vi "Write Numeric to CSV File.vi"(8 "error in (no error)":errorcluster, 9 "Time String":string, 10 "Numeric":dbl, 11 "Byte Stream File in":refnum<file>) -> (0 "error out":errorcluster, 2 "Numeric Return":dbl, 3 "Byte Stream File out":refnum<file>)   [LabVIEW 2021]
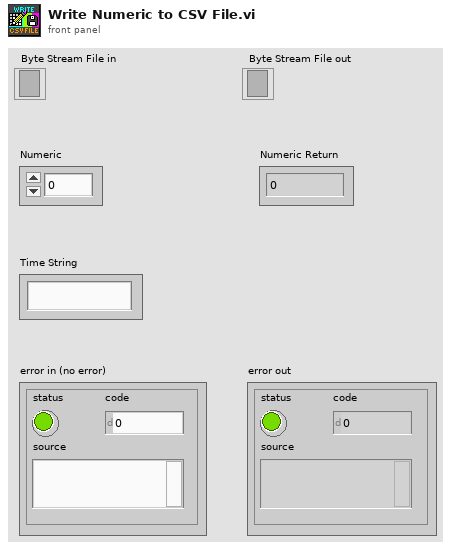
[diagram p1: front panel]
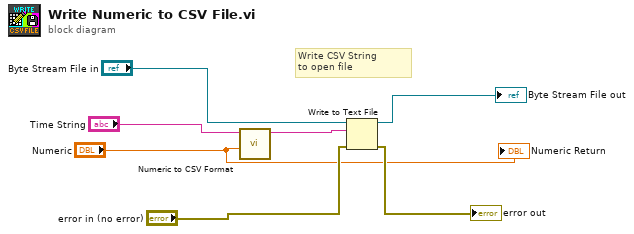
[diagram p0: block diagram]
diagram:
  # "Write CSV String\nto open file"
  n1 = call "Numeric to CSV Format.vi"("Numeric"="Numeric", "Time String"="Time String") -> ("spreadsheet string"=w3:string)  [unwired: 9 in]
  n2 = Write to Text File(file (use dialog)="Byte Stream File in", text=w3, error in="error in (no error)") -> (refnum out=→"Byte Stream File out":refnum<file>, error out=→"error out":errorcluster)  [unwired: 1 in, 1 out]
  "Numeric Return" <- "Numeric"
